vi "build_read_data_query_string.vi"() -> (3 "Query String":string)   [LabVIEW 2025, in "Newtons4thEkg.lvlib"]
uses:
  Newtons4thEkg.lvlib
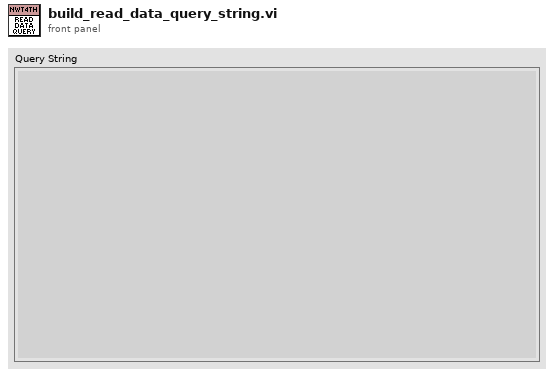
[diagram p1: front panel]
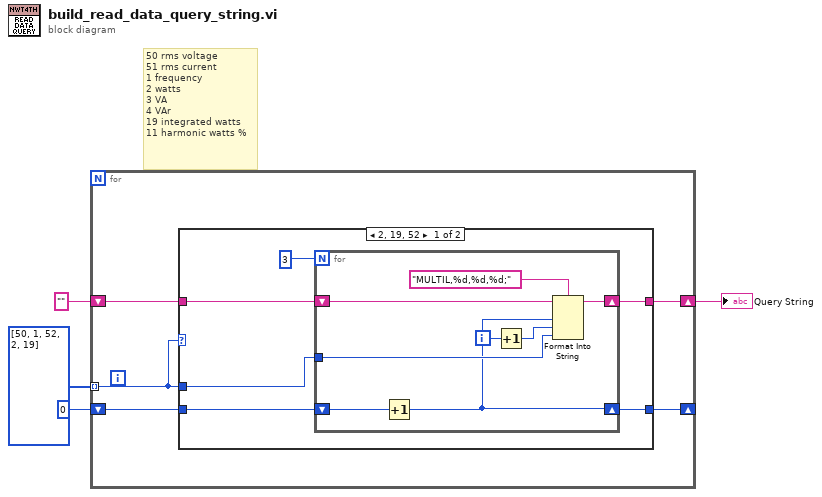
[diagram p0: block diagram]
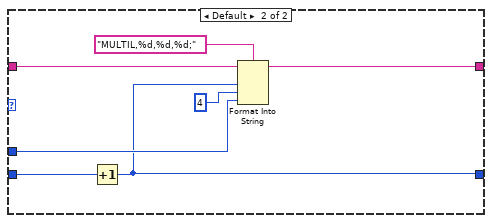
[diagram p2: hidden frame]
diagram:
  # "50 rms voltage  \n51 rms current\n1 frequency  \n2 watts  \n3 VA  \n4 VAr\n19 integrated watts\n11 harmonic watts %"
  n1 = for {
    shift-right: [w8] -> w2
    shift-left: "" -> [w9]
    tunnel: i32[] [50, 1, 52, 2, 19] -> [w7] mode=indexing
    shift-right: [w5] -> _
    shift-left: 0 -> [w6]
    n2 = case shown="2, 19, 52" w7 {
      tunnel: w9 -> [w15 w30]
      tunnel: [w14 w29] -> w8
      tunnel: w7 -> [w13 w28]
      tunnel: w6 -> [w12 w24]
      tunnel: [w10 w25] -> w5
      frame 2, 19, 52 {
        n3 = for {
          N: 3 -> [_]
          tunnel: w13 -> [w20]
          shift-right: [w21] -> w14
          shift-left: w15 -> [w22]
          shift-right: [w16] -> w10
          shift-left: w12 -> [w19]
          i -> [w18]
          n4 = Increment(x=w19) -> (x+1=w16:i32)
          n5 = Increment(x=w18) -> (x+1=w17:i32)
          n6 = Format Into String(format string="MULTIL,%d,%d,%d;", initial string=w22, w16, w17, w20) -> (resulting string=w21:string)  [unwired: 1 in, 1 out]
        }
      }
      frame Default {
        n7 = Increment(x=w24) -> (x+1=w25:i32)
        n8 = Format Into String(format string="MULTIL,%d,%d,%d;", initial string=w30, w25, 4 ("Numeric"), w28) -> (resulting string=w29:string)  [unwired: 1 in, 1 out]
      }
    }
  }
  "Query String" <- w2
